vi "NIIE_GetComparisonResult4Graphis.vi"(7 "AND Vs OR":bool, 11 "results":T1) -> (3 "True? Out":bool)   [LabVIEW 2021]
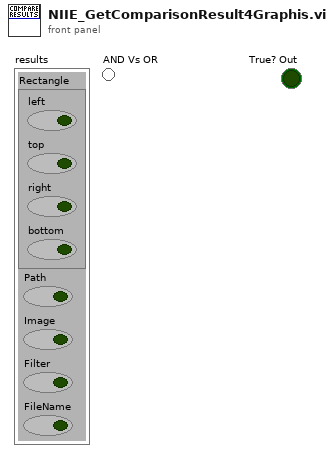
[diagram p1: front panel]
types:
  T1 = cluster{"Rectangle":cluster{"left":bool, "top":bool, "right":bool, "bottom":bool}, "Path":bool, "Image":bool, "Filter":bool, "FileName":bool}
  T2 = cluster{"left":bool, "top":bool, "right":bool, "bottom":bool}
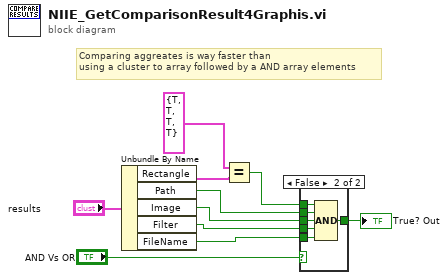
[diagram p0: block diagram]
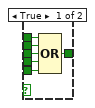
[diagram p2: hidden frame]
diagram:
  # "Comparing aggreates is way faster than\nusing a cluster to array followed by a AND array elements"
  n1 = Unbundle By Name("results") -> ("Rectangle"=w4:T2, "Path"=w7:bool, "Image"=w8:bool, "Filter"=w9:bool, "FileName"=w10:bool)
  n2 = Equal?(x=T2 {"left"=TRUE, "top"=TRUE, "right"=TRUE, "bottom"=TRUE} ("Rectangle"), y=w4) -> (x = y?=w2:bool)
  n3 = case shown="False" "AND Vs OR" {
    tunnel: w10 -> [w16 w22]
    tunnel: w9 -> [w15 w21]
    tunnel: w8 -> [w14 w20]
    tunnel: w7 -> [w13 w19]
    tunnel: w2 -> [w12 w18]
    tunnel: [w11 w17] -> w6
    frame True {
      n4 = Compound Arithmetic op=OR(w12, w13, w14, w15, w16) -> (w11:bool)
    }
    frame False {
      n5 = Compound Arithmetic op=AND(w18, w19, w20, w21, w22) -> (w17:bool)
    }
  }
  "True? Out" <- w6
